vi "Configure Root Folder.vi"(8 "Error In":errorcluster, 11 "Root Folder":path) -> (0 "Error Out":errorcluster)   [LabVIEW 2017, in "Toolkit.lvlib"]
doc: "Sets the location for creating the default log file and any rollover log files."
uses:
  Toolkit.lvlib
  Support VIs/File/Action.ctl
  Support VIs/File/File.lvlib
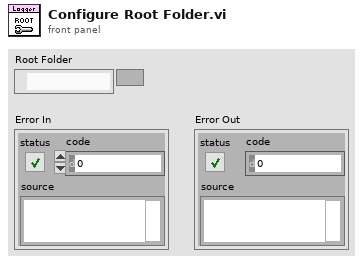
[diagram p1: front panel]
types:
  T1 = typedef "Toolkit.lvlib/File.lvlib/Action.ctl" = enum16{"Initialize", "Set Maximum File Size", "Set Maximum File Count", "Set Root Folder", "Set Enable Calendar Folder Tree", "Set File Extension", "Start", "Write", "Stop", "Shutdown"}
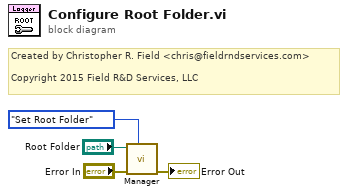
[diagram p0: block diagram]
diagram:
  # "Created by Christopher R. Field <chris@fieldrndservices.com>\n\nCopyright 2015 Field R&D Services, LLC"
  n1 = call "Manager.vi"("Action"=Action."Set Root Folder", "Error In"="Error In", "Set Value"="Root Folder") -> ("Error Out"=→"Error Out":errorcluster)  [unwired: 8 in]
